vi "Get List of Requirements.vi"(8 "error in (no error)":errorcluster, 10 "Filter":T1, 11 "Pips in":refnum<class "Pips.lvclass">) -> (0 "error out":errorcluster, 2 "RequirementIDs":string[](array[string]), 3 "Pips out":refnum<class "Pips.lvclass">)   [LabVIEW 2021, in "Bananas.lvlib" / "Pips.lvclass"]
uses:
  Pips.lvclass
  pip_filter -- enum.ctl
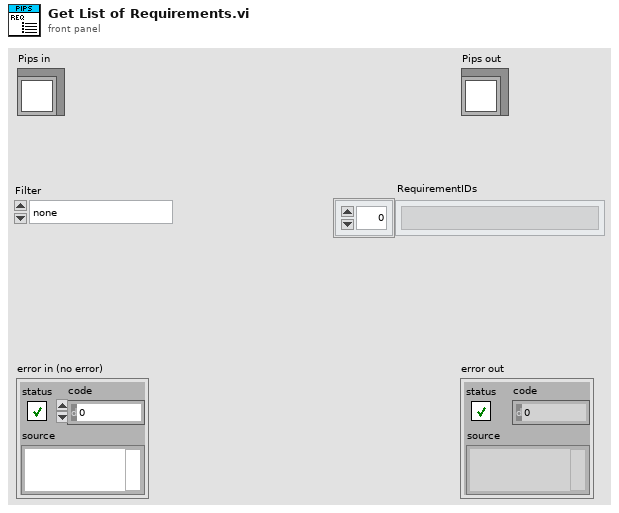
[diagram p1: front panel]
types:
  T1 = typedef "pip_filter -- enum.ctl" = enum16{"none", "passed", "skipped", "covered", "uncovered"}
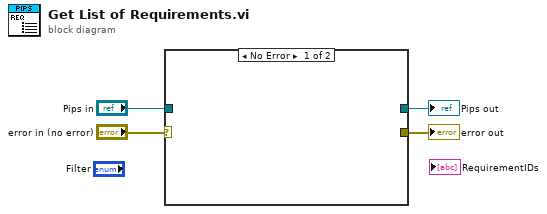
[diagram p0: block diagram]
diagram:
  n1 = case shown="No Error" "error in (no error)" {
    selector: "error in (no error)" -> [_ w6]
    tunnel: [_ w6] -> w3
    tunnel: [_ w5] -> w1
    tunnel: "Pips in" -> [_ w5]
    frame No Error {
    }
    frame Error {
    }
  }
  "error out" <- w3
  "Pips out" <- w1
